vi "main -不同数据类型.vi"() -> ()   [LabVIEW 2018]
uses:
  <vilib>/Instr/_visa.llb/VISA Configure Serial Port (Instr).vi
panel:
  out "波形图表 2":i32(graph)
  out "子字符串之后":string
  out "波形图表":i32(graph)
  out "Serial flag":bool
  out "枚举":T1
  in  "baud rate":u64(ring) items=["9600"=9600, "14400"=14400, "115200"=115200]
  out "read buffer":string
  out "serial_state":bool
  in  "serial":refnum<visa-resource-name> caption="serial_select"
  in  "serial_open":bool
  in  "exit":bool
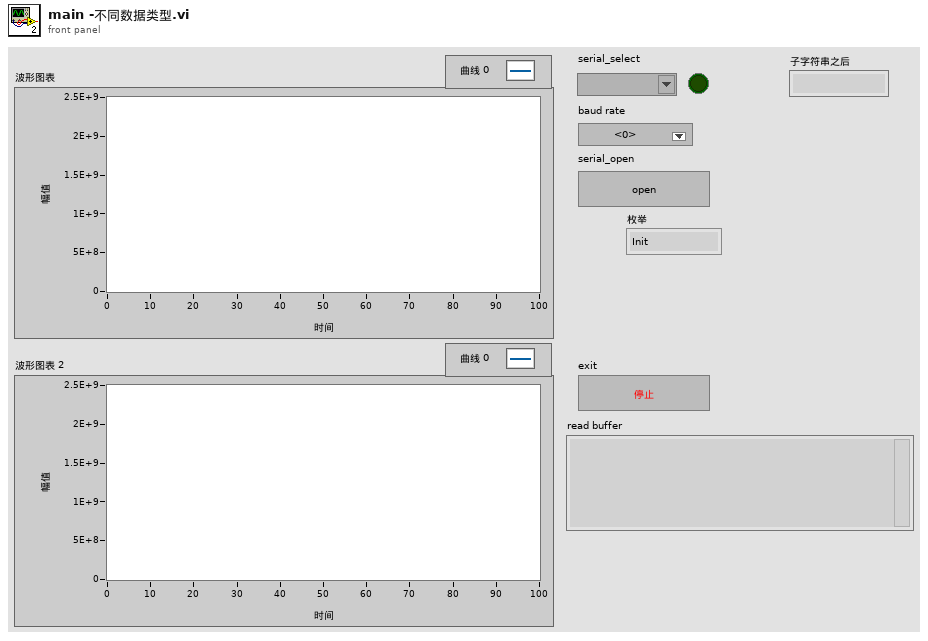
[diagram p1: front panel]
types:
  T1 = typedef "状态机.ctl" = enum16{"Init", "Send", "Wait", "GetData", "Deal", "Exit"}
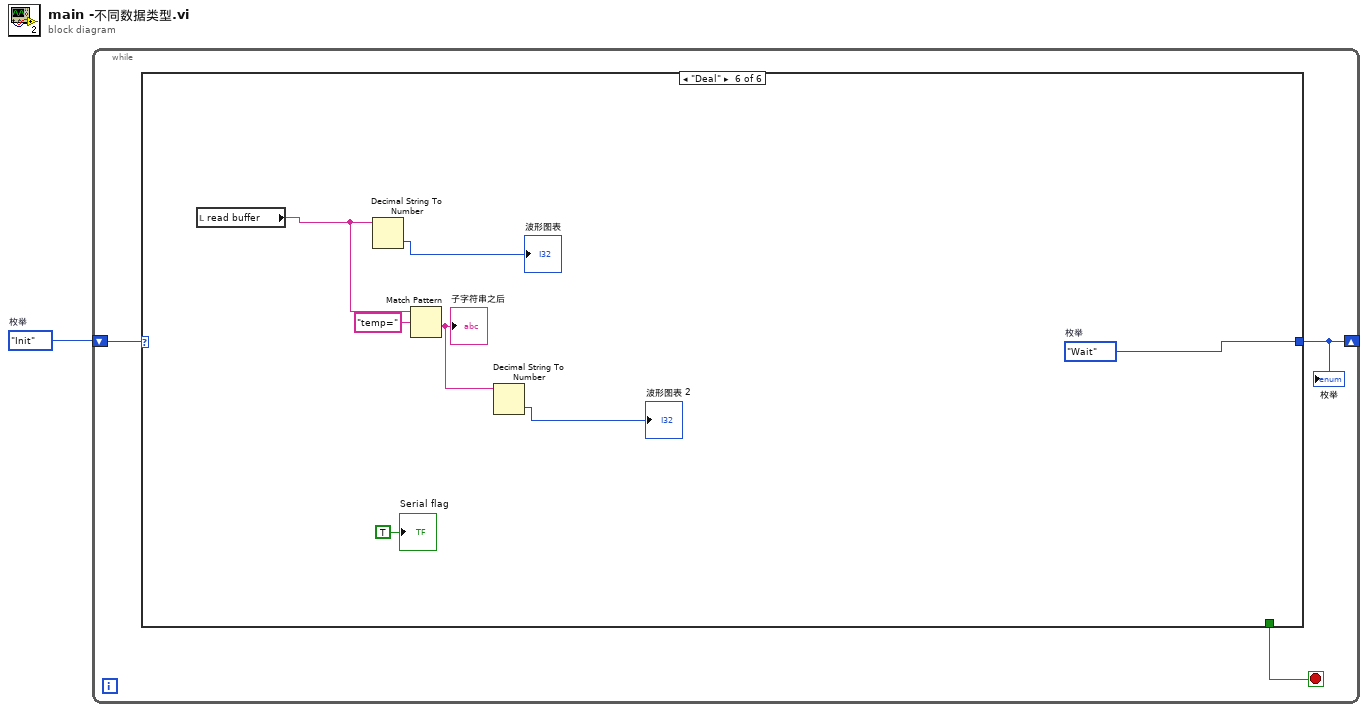
[diagram p0: block diagram]
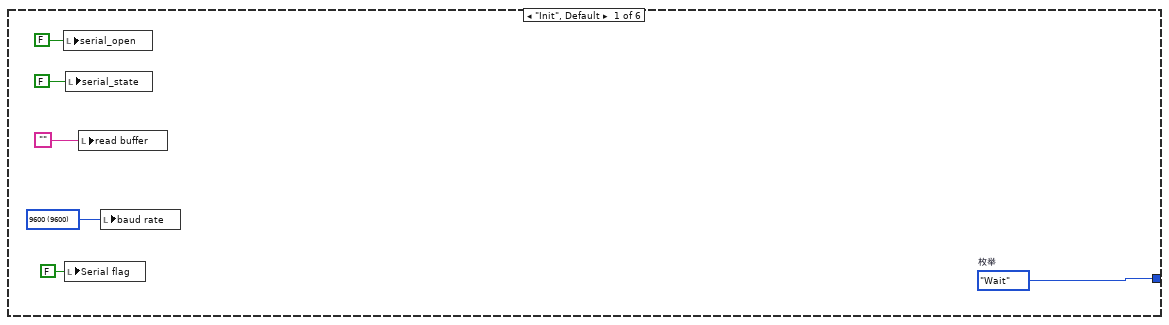
[diagram p2: hidden frame]
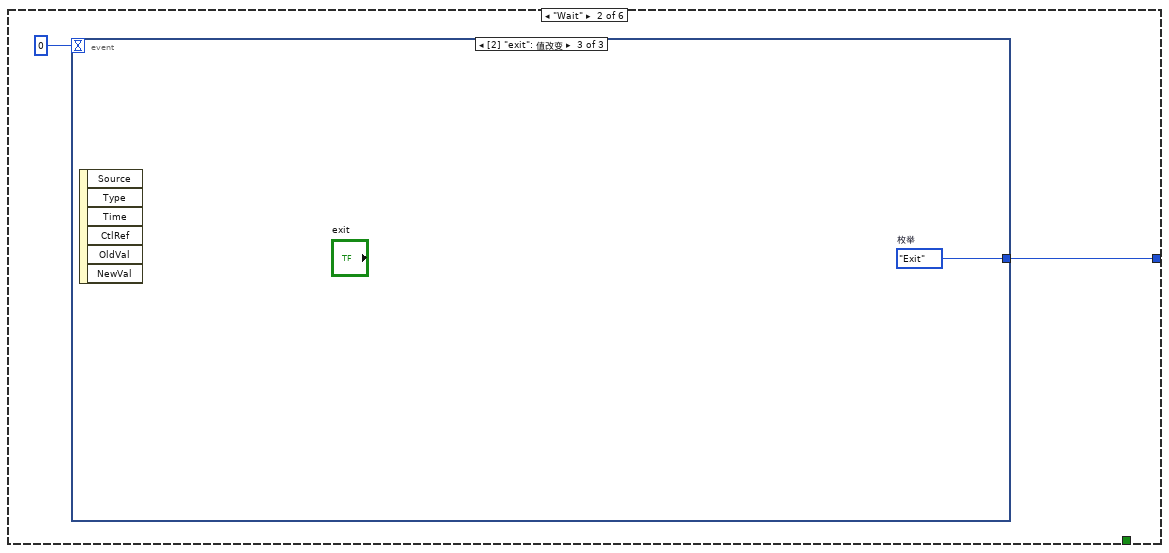
[diagram p3: hidden frame]
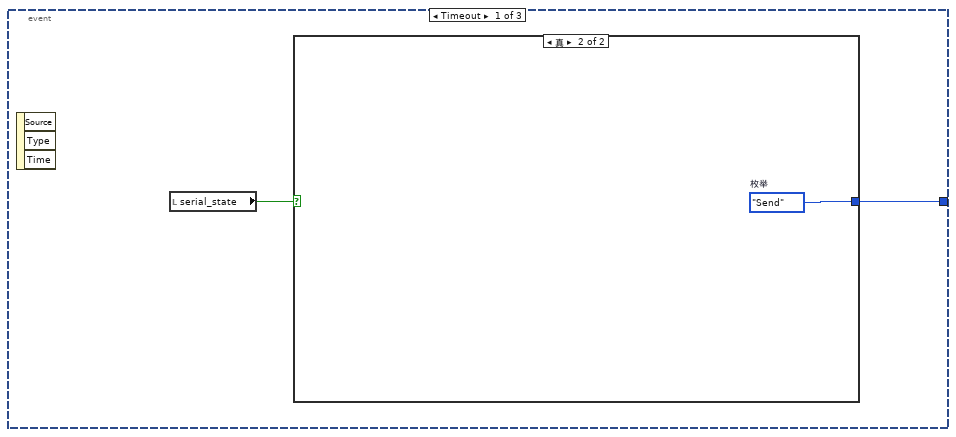
[diagram p4: hidden frame]
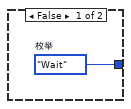
[diagram p5: hidden frame]
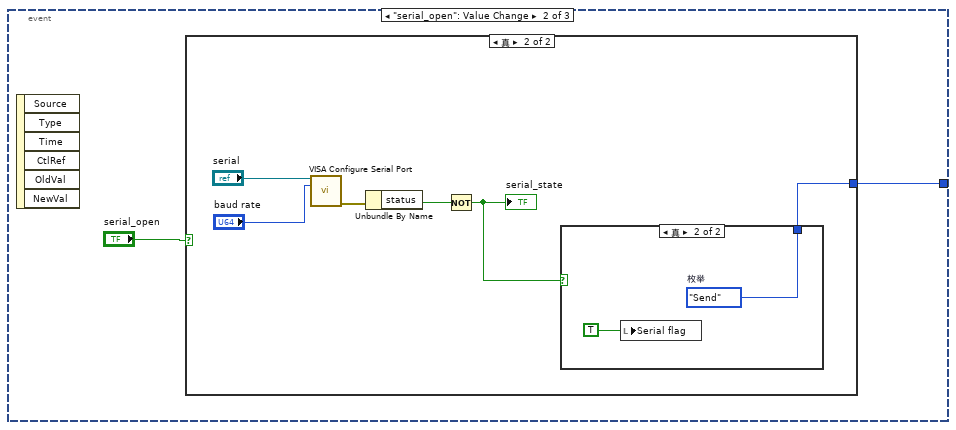
[diagram p6: hidden frame]
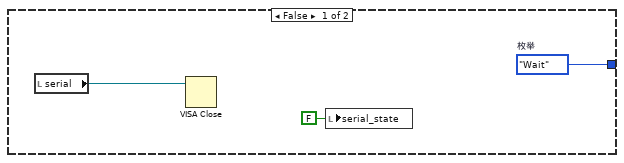
[diagram p7: hidden frame]
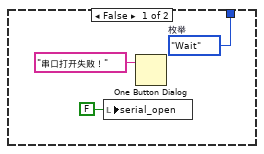
[diagram p8: hidden frame]
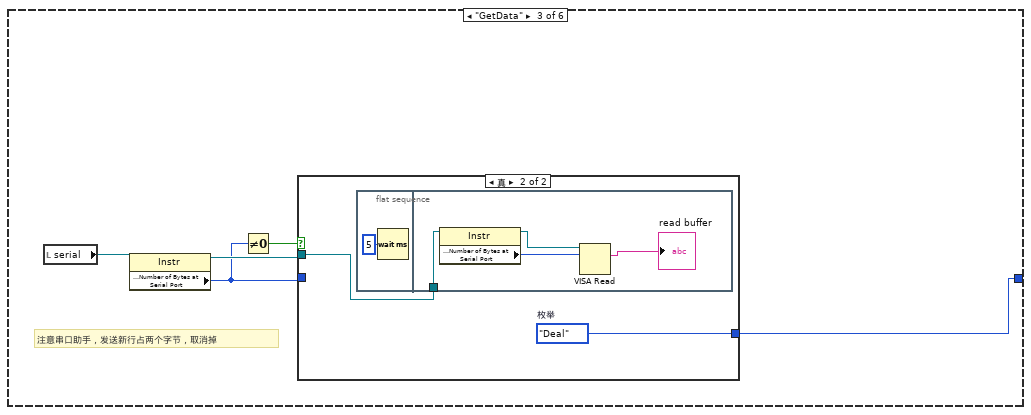
[diagram p9: hidden frame]
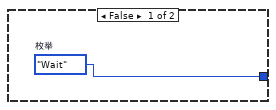
[diagram p10: hidden frame]
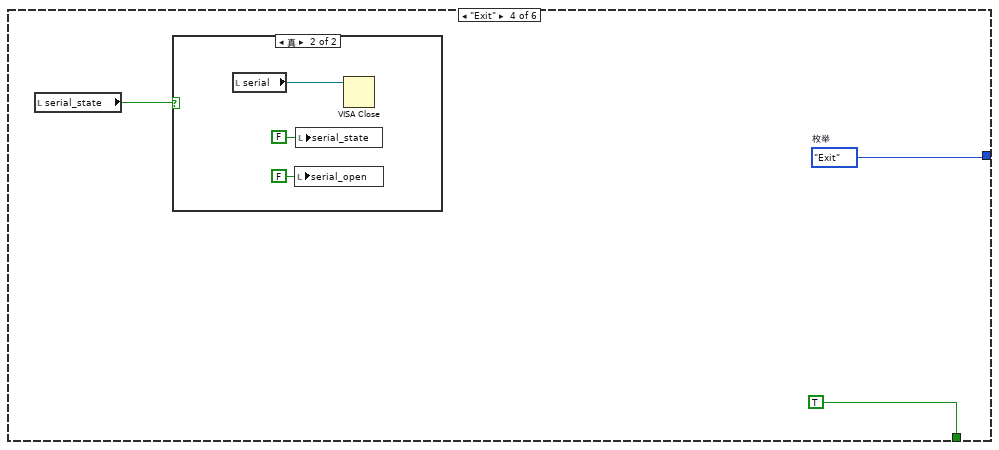
[diagram p11: hidden frame]
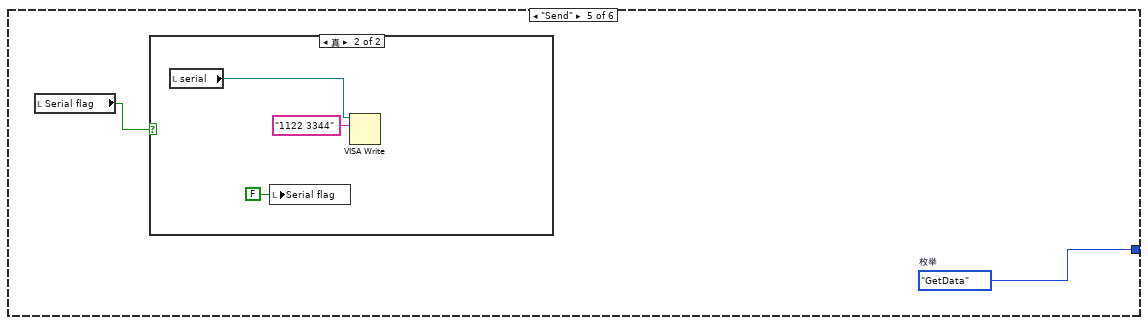
[diagram p13: hidden frame]
diagram:
  w1 = 状态机."Init"  # 枚举
  n1 = while {
    shift-right: [w3] -> _
    shift-left: w1 -> [w4]
    stop <- w2 stop-if-true
    n2 = case shown="\"Deal\"" w4 {
      tunnel: [w8 w11 w34 w49 w53 w64] -> w3
      tunnel: [_ _ _ TRUE _ _] -> w2
      frame "Init", Default {
        w6 = u64 9600 items=["9600"=9600, "115200"=115200] ("baud rate")
        w8 = 状态机."Wait"  # 枚举
        n3 = local write "serial_open"(FALSE ("serial_open")) -> ()
        n4 = local write "Serial flag"(FALSE ("Serial flag")) -> ()
        n5 = local write "serial_state"(FALSE ("serial_state")) -> ()
        n6 = local write "read buffer"("") -> ()
        n7 = local write "baud rate"(w6) -> ()
      }
      frame "Wait" {
        n8 = event shown="[2] \"exit\": 值改变" {
          selector: _ -> [_ _ _]
          dyn-events: _ -> [_ _ _]
          timeout: 0 -> [_ _ _]
          tunnel: [w13 w17 w33] -> w11
          event Timeout {
            n9 = event-data() -> ()  [unwired: 1 in, 3 out]
            n10 = local read "serial_state"() -> (w14:bool)
            n11 = case shown="真" w14 {
              tunnel: [w15 w16] -> w13
              frame False {
                w15 = 状态机."Wait"  # 枚举
              }
              frame True {
                w16 = 状态机."Send"  # 枚举
              }
            }
          }
          event "serial_open": Value Change {
            n12 = event-data() -> ()  [unwired: 1 in, 6 out]
            n13 = case shown="真" "serial_open" {
              tunnel: [w19 w23] -> w17
              frame False {
                w19 = 状态机."Wait"  # 枚举
                n14 = local read "serial"() -> (w21:refnum<visa-resource-name>)
                n15 = VISA Close(VISA resource name=w21) -> ()  [unwired: 1 in, 1 out]
                n16 = local write "serial_state"(FALSE ("serial_state")) -> ()
              }
              frame True {
                n17 = call-poly "VISA Configure Serial Port"("VISA resource name"="serial", "baud rate (9600)"="baud rate") -> ("error out"=w26:errorcluster)  [unwired: 12 in, 1 out]
                n18 = Unbundle By Name(w26) -> ("status"=w25:bool)
                n19 = Not(x=w25) -> (.not. x?=w24:bool)
                "serial_state" <- w24
                n20 = case shown="真" w24 {
                  tunnel: [w28 w32] -> w23
                  frame False {
                    w28 = 状态机."Wait"  # 枚举
                    n21 = local write "serial_open"(FALSE ("serial_open")) -> ()
                    n22 = One Button Dialog(message="串口打开失败！" ("消息")) -> ()  [unwired: 1 in, 1 out]
                  }
                  frame True {
                    w32 = 状态机."Send"  # 枚举
                    n23 = local write "Serial flag"(TRUE ("Serial flag")) -> ()
                  }
                }
              }
            }
          }
          event "exit": Value Change {
            w33 = 状态机."Exit"  # 枚举
            n24 = event-data() -> ()  [unwired: 1 in, 6 out]
          }
        }
      }
      frame "GetData" {
        # "注意串口助手，发送新行占两个字节，取消掉"
        n25 = local read "serial"() -> (w35:refnum<visa-resource-name>)
        n26 = property class="Instr"(reference=w35) -> (reference out=w38:refnum<visa-resource-name>, "Serial Settings:Number of Bytes at Serial Port"=w36:u32)  [unwired: 1 in, 1 out]
        n27 = Not Equal To 0?(x=w36) -> (x != 0?=w37:bool)
        n28 = case shown="真" w37 {
          tunnel: w38 -> [_ w40]
          tunnel: w36 -> [_ _]
          tunnel: [w39 w41] -> w34
          frame False {
            w39 = 状态机."Wait"  # 枚举
          }
          frame True {
            w41 = 状态机."Deal"  # 枚举
            n29 = flat-sequence {
              tunnel: w40 -> [w45]
              frame #0 {
                n30 = Wait (ms)(milliseconds to wait=u32 5 ("等待时间（毫秒）")) -> ()  [unwired: 1 out]
              }
              frame #1 {
                n31 = property class="Instr"(reference=w45) -> (reference out=w43:refnum<visa-resource-name>, "Serial Settings:Number of Bytes at Serial Port"=w44:u32)  [unwired: 1 in, 1 out]
                n32 = VISA Read(VISA resource name=w43, byte count=w44) -> (read buffer=→"read buffer":string)  [unwired: 1 in, 3 out]
              }
            }
          }
        }
      }
      frame "Exit" {
        w49 = 状态机."Exit"  # 枚举
        n33 = local read "serial_state"() -> (w47:bool)
        n34 = case shown="真" w47 {
          frame False {
          }
          frame True {
            n35 = local read "serial"() -> (w52:refnum<visa-resource-name>)
            n36 = local write "serial_open"(FALSE ("serial_state")) -> ()
            n37 = local write "serial_state"(FALSE ("serial_state")) -> ()
            n38 = VISA Close(VISA resource name=w52) -> ()  [unwired: 1 in, 1 out]
          }
        }
      }
      frame "Send" {
        w53 = 状态机."GetData"  # 枚举
        n39 = local read "Serial flag"() -> (w54:bool)
        n40 = case shown="真" w54 {
          frame False {
          }
          frame True {
            n41 = local read "serial"() -> (w56:refnum<visa-resource-name>)
            n42 = local write "Serial flag"(FALSE ("Serial flag")) -> ()
            n43 = VISA Write(VISA resource name=w56, write buffer="1122 3344" ("写入缓冲区")) -> ()  [unwired: 1 in, 3 out]
          }
        }
      }
      frame "Deal" {
        w64 = 状态机."Wait"  # 枚举
        n44 = local read "read buffer"() -> (w61:string)
        n45 = Decimal String To Number(string=w61) -> (number=→"波形图表":i32)  [unwired: 2 in, 1 out]
        n46 = Match Pattern(string=w61, regular expression="temp=" ("正则表达式")) -> (after substring=w58:string)  [unwired: 1 in, 3 out]
        "子字符串之后" <- w58
        n47 = Decimal String To Number(string=w58) -> (number=→"波形图表 2":i32)  [unwired: 2 in, 1 out]
        "Serial flag" <- TRUE ("Serial flag")
      }
    }
    "枚举" <- w3
  }
